vi "DriveHalt.vi"(1 "Parameter String":string, 2 "Reinit":bool) -> (0 "Increment":bool)   [LabVIEW 2018]
uses:
  instructions.vi
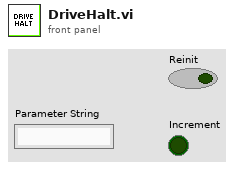
[diagram p1: front panel]
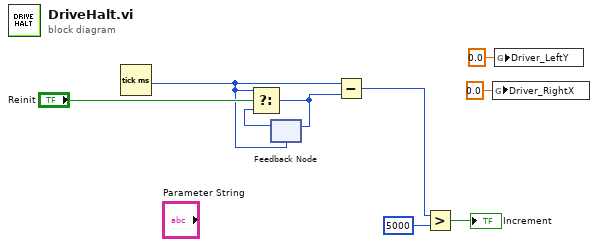
[diagram p0: block diagram]
diagram:
  n1 = Tick Count (ms)() -> (millisecond timer value=w2:u32)
  n2 = feedback #1(w2) -> (w8:u32)
  n3 = Select(t=w2, s="Reinit", f=w8) -> (s? t:f=w6:u32)
  n4 = feedback-in #1(w6) -> ()
  n5 = Subtract(x=w2, y=w6) -> (x-y=w5:u32)
  n6 = Greater?(x=w5, y=u32 5000) -> (0:→"Increment":bool)
  n7 = global write "instructions.vi" "Driver_RightX"(0.0 ("Driver_RightX")) -> ()
  n8 = global write "instructions.vi" "Driver_LeftY"(0.0 ("Driver_LeftY")) -> ()
